vi "Archive User.vi"(11 "REFERENCES":T1) -> ()   [LabVIEW 2019]
uses:
  Controls/References Cluster.ctl
  Controls/Custom Calendar/Custom Calendar.xctl
  Controls/Table Data Types/User Data Type.ctl
  Controls/Table Data Types/User Archive Data Type.ctl
  <vilib>/addons/database/Connection.llb/DB Tools Open Connec (String).vi
  <vilib>/addons/database/_DB Variant To Data/Database Variant To Data.xnode
  <vilib>/addons/database/NI_Database_API.lvlib
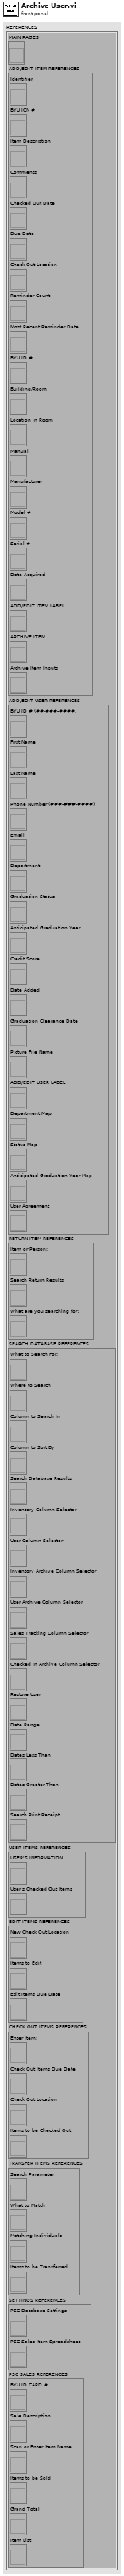
[diagram p1: front panel]
types:
  T1 = typedef "References Cluster.ctl" = cluster{"MAIN PAGES":refnum<vi>, "ADD/EDIT ITEM REFERENCES":cluster{"Identifier":refnum<vi>, "BYU ICN #":refnum<vi>, "Item Description":refnum<vi>, "Comments":refnum<vi>, "Checked Out Date":refnum<vi>, "Due Date":refnum<vi>, "Check Out Location":refnum<vi>, "Reminder Count":refnum<vi>, "Most Recent Reminder Date":refnum<vi>, "BYU ID #":refnum<vi>, "Building/Room":refnum<vi>, "Location in Room":refnum<vi>, "Manual":refnum<vi>, "Manufacturer":refnum<vi>, "Model #":refnum<vi>, "Serial #":refnum<vi>, "Date Acquired":refnum<vi>, "ADD/EDIT ITEM LABEL":refnum<vi>, "ARCHIVE ITEM":refnum<vi>, "Archive Item Inputs":refnum<vi>}, "ADD/EDIT USER REFERENCES":cluster{"BYU ID # (##-###-####)":refnum<vi>, "First Name":refnum<vi>, "Last Name":refnum<vi>, "Phone Number (###-###-####)":refnum<vi>, "Email":refnum<vi>, "Department":refnum<vi>, "Graduation Status":refnum<vi>, "Anticipated Graduation Year":refnum<vi>, "Credit Score":refnum<vi>, "Date Added":refnum<vi>, "Graduation Clearance Date":refnum<vi>, "Picture File Name":refnum<vi>, "ADD/EDIT USER LABEL":refnum<vi>, "Department Map":refnum<vi>, "Status Map":refnum<vi>, "Anticipated Graduation Year Map":refnum<vi>, "User Agreement":refnum<vi>}, "RETURN ITEM REFERENCES":cluster{"Item or Person:":refnum<vi>, "Search Return Results":refnum<vi>, "What are you searching for?":refnum<vi>}, "SEARCH DATABASE REFERENCES":cluster{"What to Search For:":refnum<vi>, "Where to Search":refnum<vi>, "Column to Search In":refnum<vi>, "Column to Sort By":refnum<vi>, "Search Database Results":refnum<vi>, "Inventory Column Selector":refnum<vi>, "User Column Selector":refnum<vi>, "Inventory Archive Column Selector":refnum<vi>, "User Archive Column Selector":refnum<vi>, "Sales Tracking Column Selector":refnum<vi>, "Checked In Archive Column Selector":refnum<vi>, "Restore User":refnum<vi>, "Date Range":refnum<vi>, "Dates Less Than":refnum<vi>, "Dates Greater Than":refnum<vi>, "Search Print Receipt":refnum<vi>}, "USER ITEMS REFERENCES":cluster{"USER'S INFORMATION":refnum<vi>, "User's Checked Out Items":refnum<vi>}, "EDIT ITEMS REFERENCES":cluster{"New Check Out Location":refnum<vi>, "Items to Edit":refnum<vi>, "Edit Items Due Date":refnum<vi>}, "CHECK OUT ITEMS REFERENCES":cluster{"Enter Item:":refnum<vi>, "Check Out Items Due Date":refnum<vi>, "Check Out Location":refnum<vi>, "Items to be Checked Out":refnum<vi>}, "TRANSFER ITEMS REFERENCES":cluster{"Search Parameter":refnum<vi>, "What to Match":refnum<vi>, "Matching Individuals":refnum<vi>, "Items to be Transferred":refnum<vi>}, "SETTINGS REFERENCES":cluster{"PSC Database Settings":refnum<vi>, "PSC Sales Item Spreadsheet":refnum<vi>}, "PSC SALES REFERENCES":cluster{"BYU ID CARD #":refnum<vi>, "Sale Description":refnum<vi>, "Scan or Enter Item Name":refnum<vi>, "Items to be Sold":refnum<vi>, "Grand Total":refnum<vi>, "Item List":refnum<vi>}}
  T2 = typedef "User Archive Data Type.ctl" = cluster{"BYU ID #":string, "First Name":string, "Last Name":string, "Phone Number":string, "Email":string, "Department":string, "Graduation Status":string, "Anticipated Graduation Year":string, "Credit Score":dbl, "Date Added":string, "Graduation Clearance Date":string, "Picture File Name":string, "Date Archived":string}
  T3 = typedef "User Data Type.ctl" = cluster{"BYU ID #":string, "First Name":string, "Last Name":string, "Phone Number":string, "Email":string, "Department":string, "Graduation Status":string, "Anticipated Graduation Year":string, "Credit Score":dbl, "Date Added":string, "Graduation Clearance Date":string, "Picture File Name":string}
  T4 = cluster{"USER'S INFORMATION":refnum<vi>, "User's Checked Out Items":refnum<vi>}
  T5 = typedef "IMAQ Image.ctl" = refnum<image>
  T6 = cluster{"BYU ID #":string, "First Name":string, "Last Name":string, "Phone":string, "Email":string, "Department":string, "Status":string, "Grad Year":string, "Date Added":string, "Grad Clearance Date":string, "Credit Score":string, "User Items Photo":T5}
  T7 = typedef "NI_Database_API.lvlib/Conn ObjectReference.ctl" = refnum<k1>
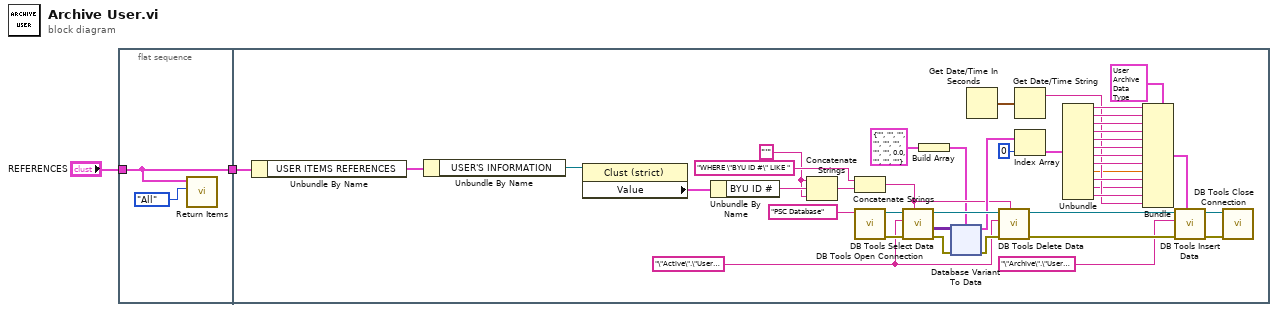
[diagram p0: block diagram]
diagram:
  n1 = flat-sequence {
    tunnel: "REFERENCES" -> [w3]
    tunnel: [w3] -> w1
    tunnel: w1 -> [w16]
    frame #0 {
      n2 = call "Return Items.vi"("Selection"=enum16{"Selection", "All"}."All", "REFERENCES"=w3) -> ()  [unwired: 10 in]
    }
    frame #1 {
      w5 = "'" ("string")
      w23 = "\"Active\".\"Users\""
      n3 = Unbundle By Name(w16) -> ("USER ITEMS REFERENCES"=w15:T4)
      n4 = Unbundle By Name(w15) -> ("USER'S INFORMATION"=w47:refnum<vi>)
      n5 = property class="Clust (strict)"(reference=w47) -> ("Value"=w14:T6)  [unwired: 1 in, 2 out]
      n6 = Unbundle By Name(w14) -> ("BYU ID #"=w6:string)
      n7 = Concatenate Strings(w5, w6, w5) -> (w7:string)
      n8 = Concatenate Strings("WHERE \"BYU ID #\" LIKE " ("string"), w7) -> (w24:string)
      n9 = call-poly <vilib>:"DB Tools Open Connection.vi"("connection information"="PSC Database") -> ("error out"=w44:errorcluster, "connection reference"=w45:T7)  [unwired: 7 in]
      n10 = call <vilib>:"DB Tools Select Data.vi"("condition"=w24, "error in (no error)"=w44, "table"=w23, "connection reference"=w45) -> ("error out"=w41:errorcluster, "data"=w42:variant[][], "connection reference out"=w43:T7)  [unwired: 2 in]
      n11 = Build Array(T3 {"BYU ID #"="", "First Name"="", "Last Name"="", "Phone Number"="", "Email"="", "Department"="", "Graduation Status"="", "Anticipated Graduation Year"="", "Credit Score"=0.0, "Date Added"="", "Graduation Clearance Date"="", "Picture File Name"=""} ("Array")) -> (w12:T3[])
      n12 = xnode "Database Variant To Data"("database variant"=w42, "error in (no error)"=w41, "type"=w12) -> ("data"=w39:T3[], "error out"=w40:errorcluster)
      n13 = Get Date/Time In Seconds() -> (seconds since 1Jan1904=w26:timestamp)
      n14 = call <vilib>:"DB Tools Delete Data.vi"("condition"=w24, "error in (no error)"=w40, "table"=w23, "connection reference"=w43) -> ("error out"=w20:errorcluster, "connection reference out"=w21:T7)  [unwired: 6 in]
      n15 = Get Date/Time String(seconds (now)=w26) -> (date string=w25:string)  [unwired: 2 in, 1 out]
      n16 = Index Array(array=w39, index=0) -> (element=w37:T3)
      n17 = Unbundle(w37) -> ("BYU ID #"=w36:string, "First Name"=w35:string, "Last Name"=w34:string, "Phone Number"=w33:string, "Email"=w32:string, "Department"=w31:string, "Graduation Status"=w30:string, "Anticipated Graduation Year"=w29:string, "Credit Score"=w10:dbl, "Date Added"=w28:string, "Graduation Clearance Date"=w9:string, "Picture File Name"=w27:string)
      n18 = Bundle(cluster=T2 {"BYU ID #"="", "First Name"="", "Last Name"="", "Phone Number"="", "Email"="", "Department"="", "Graduation Status"="", "Anticipated Graduation Year"="", "Credit Score"=0.0, "Date Added"="", "Graduation Clearance Date"="", "Picture File Name"="", "Date Archived"=""} ("USER ARCHIVE DATA TYPE"), "BYU ID #"=w36, "First Name"=w35, "Last Name"=w34, "Phone Number"=w33, "Email"=w32, "Department"=w31, "Graduation Status"=w30, "Anticipated Graduation Year"=w29, "Credit Score"=w10, "Date Added"=w28, "Graduation Clearance Date"=w9, "Picture File Name"=w27, "Date Archived"=w25) -> (w22:T2)
      n19 = call <vilib>:"DB Tools Insert Data.vi"("data"=w22, "error in (no error)"=w20, "table"="\"Archive\".\"Users\"", "connection reference"=w21) -> ("error out"=w17:errorcluster, "connection reference out"=w18:T7)  [unwired: 6 in]
      n20 = call <vilib>:"DB Tools Close Connection.vi"("error in (no error)"=w17, "connection reference"=w18) -> ()  [unwired: 5 in, 1 out]
    }
  }
